vi "1_show_current_time.vi"() -> ()   [LabVIEW 2018]
panel:
  in  "stop":bool
  out "current time":timestamp
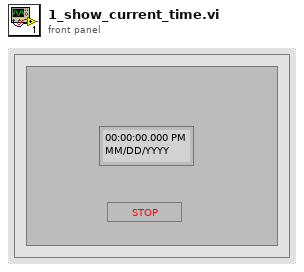
[diagram p1: front panel]
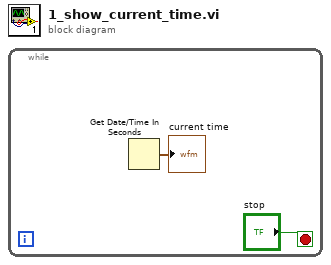
[diagram p0: block diagram]
diagram:
  n1 = while {
    stop <- "stop" stop-if-true
    n2 = Get Date/Time In Seconds() -> (seconds since 1Jan1904=→"current time":timestamp)
  }
